vi "Magnitude Square of Complex Number scalable.vi"(2 "output type":fxp<+,37,2> format="%.36g", 5 "Real":fxp<+/-,24,3>, 7 "Imaginary":fxp<+/-,24,3>, 9 "Input Valid":bool=TRUE) -> (6 "Magnitude^2":fxp<+,37,2> format="%.36g", 10 "Output Valid":bool)   [LabVIEW 2011]
doc: "This VI computes the magnitude of a complex number using two DSP48E blocks in cascade fashion.\n\n<b> Latency = 6 Ticks </b>"
uses:
  <vilib>/rvi/FXPMathLib/basic elements/FxpDiscreteDelay/XNode/nifxpmath_DiscreteDelay.xnode
  <vilib>/rvi/FXPMathLib/FxpMul/XNode/nifxpmath_Multiplier.xnode
  <vilib>/rvi/FXPMathLib/FxpInterpret/XNode/nifxpmath_Interpret.xnode
  <vilib>/rvi/FXPMathLib/sim/FxpSim.dll
panel:
  out "output type":fxp<+/-,49,7> format="%.45g"
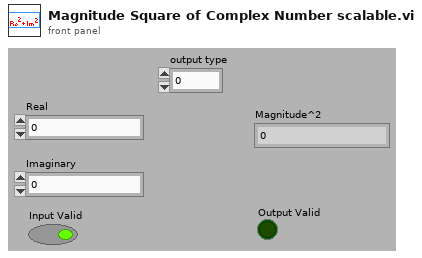
[diagram p1: front panel]
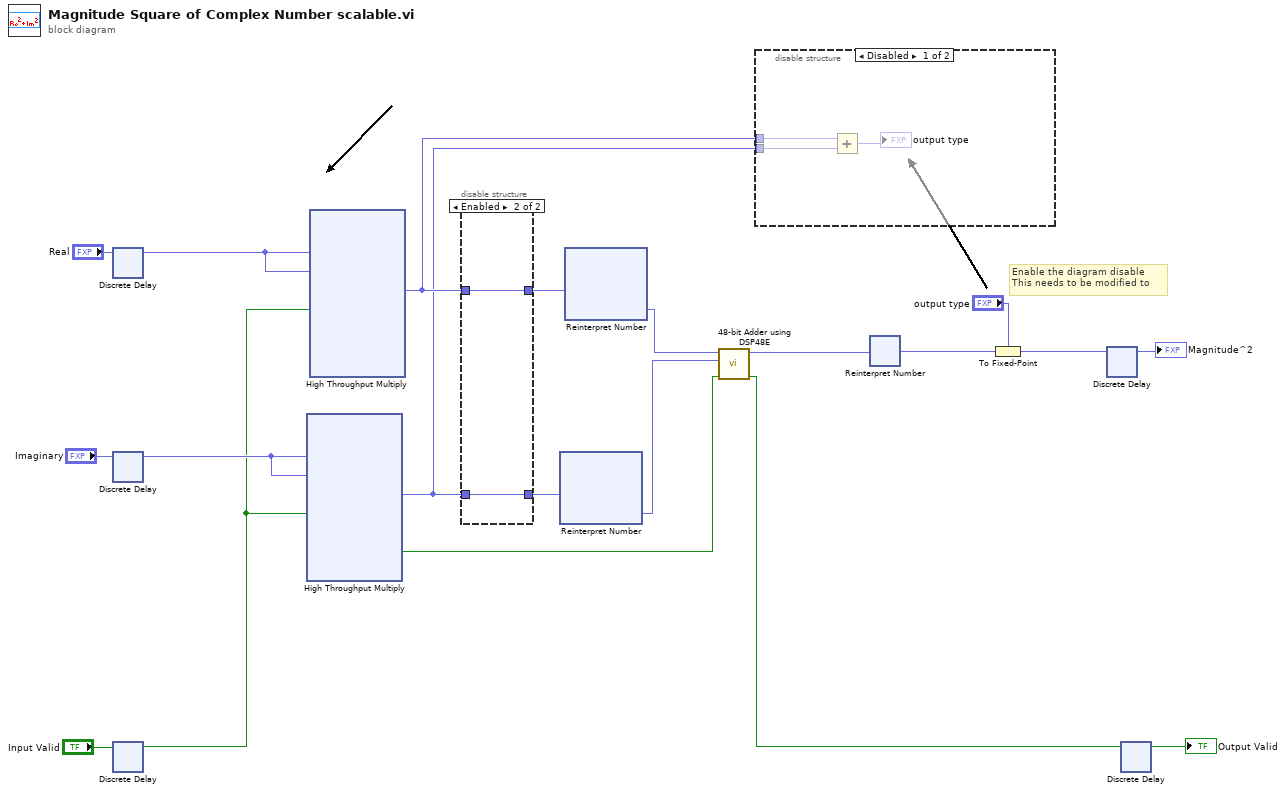
[diagram p0: block diagram]
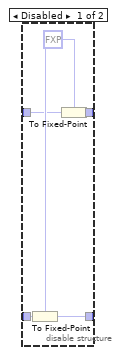
[diagram p2: hidden frame]
diagram:
  # "Enable the diagram disable\nThis needs to be modified to"
  n1 = xnode "Discrete Delay"("D"="Real") -> ("Q"=w15:fxp<+/-,24,3>)
  n2 = xnode "Discrete Delay"("D"="Imaginary") -> ("Q"=w14:fxp<+/-,24,3>)
  n3 = xnode "Discrete Delay"("D"="Input Valid") -> ("Q"=w13:bool)
  n4 = xnode "High Throughput Multiply"("x"=w14, "y"=w14, "input valid"=w13) -> ("x*y"=w11:fxp<+/-,48,6>, "output valid"=w2:bool)  [unwired: 1 in, 1 out]
  n5 = xnode "High Throughput Multiply"("x"=w15, "y"=w15, "input valid"=w13) -> ("x*y"=w12:fxp<+/-,48,6>)  [unwired: 1 in, 2 out]
  n6 = disable-structure shown="Enabled" {
    disable-tunnel: w12 -> [w24 w27]
    disable-tunnel: w11 -> [w23 w26]
    disable-tunnel: [w22 w27] -> w10
    disable-tunnel: [w21 w26] -> w9
    frame Disabled {
      w25 = fxp<+/-,48,1> 0.0 ("fixed-point type")
      n7 = To Fixed-Point(fixed-point type=w25, number=w23) -> (fixed-point=w21:fxp<+/-,48,1>)
      n8 = To Fixed-Point(fixed-point type=w25, number=w24) -> (fixed-point=w22:fxp<+/-,48,1>)
    }
    frame Enabled {
    }
  }
  n9 = xnode "Reinterpret Number"("x"=w9) -> ("y"=w8:fxp<+/-,48,48>)
  n10 = xnode "Reinterpret Number"("x"=w10) -> ("y"=w7:fxp<+/-,48,48>)
  n11 = call <userlib>:"48-bit Adder using DSP48E.vi"("Input Valid"=w2, "B"=w8, "A"=w7) -> ("Output Valid"=w1:bool, "A+B"=w6:fxp<+/-,49,49>)  [unwired: 7 in]
  n12 = disable-structure shown="Disabled" {
    disable-tunnel: w12 -> [w30 _]
    disable-tunnel: w11 -> [w29 _]
    frame Disabled {
      n13 = Add(x=w30, y=w29) -> (x+y=→"output type":fxp<+/-,49,7>)
    }
    frame Enabled {
    }
  }
  n14 = xnode "Reinterpret Number"("x"=w6) -> ("y"=w5:fxp<+/-,49,2>)
  n15 = To Fixed-Point(fixed-point type="output type", number=w5) -> (fixed-point=w4:fxp<+,37,2>)
  n16 = xnode "Discrete Delay"("D"=w4) -> ("Q"=→"Magnitude^2":fxp<+,37,2>)
  n17 = xnode "Discrete Delay"("D"=w1) -> ("Q"=→"Output Valid":bool)
